vi "Advanced Cut - Auto Forward Cut.vi"(8 "error in (no error)":errorcluster, 11 "Auto Cut (Forward)":T1={"Start Time (s)"=0.0, "# Epochs"=10, "Epoch Duration (s)"=90.0} {"Epoch Duration (s)" min=0.0 step=1.0; "Start Time (s)" min=0.0 step=1.0}) -> (0 "error out":errorcluster, 3 "Snippets":dbl[][](array[numeric]))   [LabVIEW 2016]
uses:
  Type Definitions/Advanced Cut - Forward Auto Cut.ctl
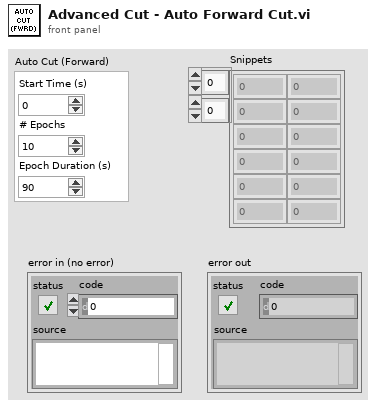
[diagram p1: front panel]
types:
  T1 = typedef "Advanced Cut - Forward Auto Cut.ctl" = cluster{"Start Time (s)":dbl, "# Epochs":u32, "Epoch Duration (s)":dbl}
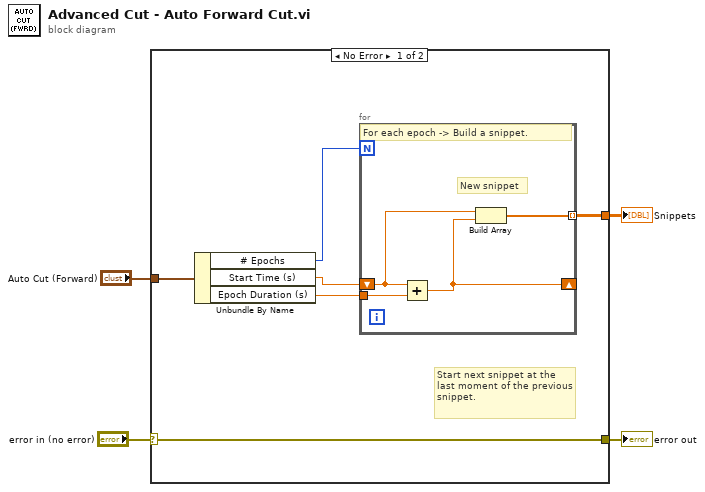
[diagram p0: block diagram]
diagram:
  n1 = case shown="No Error" "error in (no error)" {
    selector: "error in (no error)" -> [w10 w15]
    tunnel: [w10 w15] -> w3
    tunnel: [w9 _] -> w2
    tunnel: "Auto Cut (Forward)" -> [w8 _]
    frame No Error {
      # "Start next snippet at the last moment of the previous snippet."
      n2 = Unbundle By Name(w8) -> ("# Epochs"=w7:u32, "Start Time (s)"=w6:dbl, "Epoch Duration (s)"=w5:dbl)
      n3 = for {
        N: w7 -> [_]
        shift-right: [w13] -> _
        shift-left: w6 -> [w14]
        tunnel: [w12] -> w9 mode=indexing
        tunnel: w5 -> [w11]
        # "New snippet"
        # "For each epoch -> Build a snippet."
        n4 = Add(x=w14, y=w11) -> (x+y=w13:dbl)
        n5 = Build Array(w14, w13) -> (w12:dbl[])
      }
    }
    frame Error {
    }
  }
  "error out" <- w3
  "Snippets" <- w2
